vi "Stop Measurements.vi"(8 "error in (no error)":errorcluster, 11 "Pulse Controller in":refnum<class "Pulse Controller.lvclass">) -> (0 "error out":errorcluster, 3 "Pulse Controller out":refnum<class "Pulse Controller.lvclass">)   [LabVIEW 2016, in "Pulse Controller.lvclass"]
uses:
  Pulse Controller.lvclass
  C:/github/LabActor/Worker/Worker.lvclass
  C:/github/LabActor/Controllers/Process Controller/Process Controller.lvclass
  C:/github/LabActor/Template Module/Template Module.lvclass
  Worker/Worker.lvclass/Worker.ctl
  Process Controller/Process Controller.lvclass/Process Controller.ctl
  NHMFL_Core/Libraries/Instruments/Results/File Path Result/File Path Result.lvclass
  C:/github/NHMFL_Core/Libraries/Instruments/Results/Acquired Result/Acquired Result.lvclass
  Template Module/Template Module.lvclass/Template Module.ctl
  NHMFL_Core/Libraries/Instruments/Results/Acquired Result/Acquired Result.lvclass/Acquired Result.ctl
  Template Module/Read tdms stream.vi
  Template Module/Read Name.vi
  NHMFL_Core/Libraries/Instruments/Results/Acquired Result/Write Sender.vi
  Template Module/Read Reply to.vi
  Template Module/Read State.vi
  Process Controller/Read Awaiting Results.vi
  Read Pulse Controller Configuration.vi
  Template Module Messages/Result Reply Msg/Result Reply Msg.lvclass
  Process Controller/Process Controller.lvclass
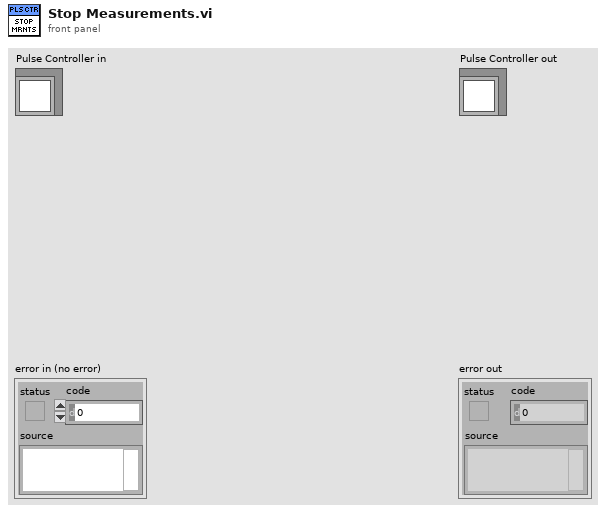
[diagram p1: front panel]
types:
  T1 = typedef "Worker State.ctl" = enum16{"Idle", "Starting", "Working", "Stopping"}
  T2 = typedef "Pulse Controller Configuration.ctl" = cluster{"Pre-trigger duration":dbl, "Post-trigger duration":dbl, "Open plot after pulse":bool}
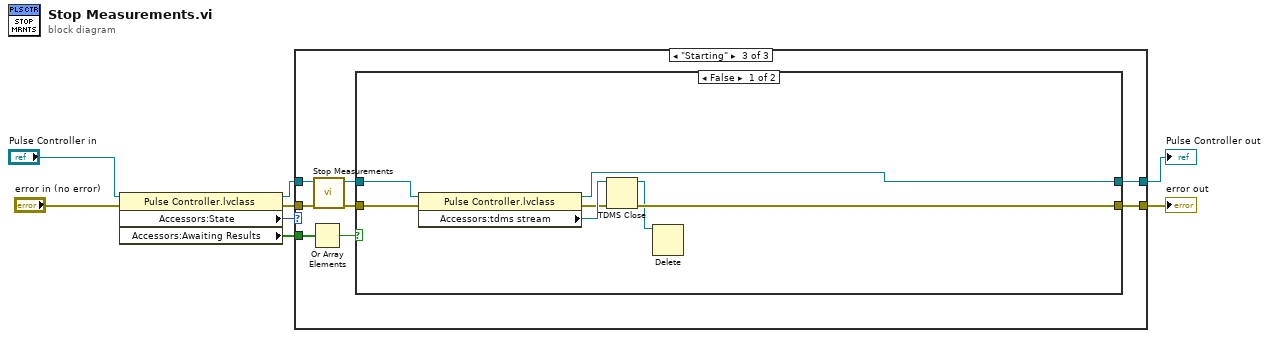
[diagram p0: block diagram]
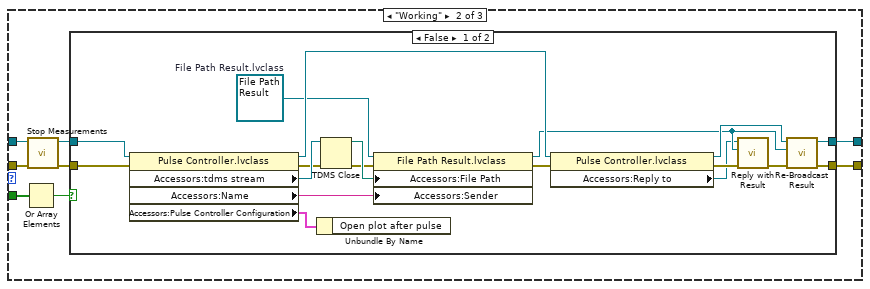
[diagram p3: hidden frame]
diagram:
  n1 = property class="Pulse Controller.lvclass"(reference="Pulse Controller in", error in="error in (no error)") -> (reference out=w3:refnum<class "Pulse Controller.lvclass">, error out=w5:errorcluster, "Accessors:State"=w2:T1, "Accessors:Awaiting Results"=w1:bool[])
  n2 = case shown="\"Starting\"" w2 {
    tunnel: w3 -> [w9 w18 w46]
    tunnel: w5 -> [w10 w14 w42]
    tunnel: [w9 w17 w45] -> w7
    tunnel: [w10 w16 w44] -> w6
    tunnel: w1 -> [_ w12 w40]
    frame "Idle", Default {
    }
    frame "Working" {
      n3 = Or Array Elements(Boolean array=w12) -> (logical OR=w11:bool)
      n4 = call-parent "Stop Measurements.vi"("error in (no error)"=w14, "Measure Controller in"=w18) -> ("error out"=w13:errorcluster, "Measure Controller out"=w15:refnum<class "Pulse Controller.lvclass">)  [unwired: 8 in]
      n5 = case shown="False" w11 {
        tunnel: [w34 w38] -> w17
        tunnel: [w23 w37] -> w16
        tunnel: w15 -> [w21 w38]
        tunnel: w13 -> [w20 w37]
        frame False {
          w31 = refnum<class "File Path Result.lvclass"> refnum  # File Path Result.lvclass
          n6 = property class="Pulse Controller.lvclass"(reference=w21, error in=w20) -> (reference out=w32:refnum<class "Pulse Controller.lvclass">, error out=w35:errorcluster, "Accessors:tdms stream"=w36:refnum<k34>, "Accessors:Name"=w26:string, "Accessors:Pulse Controller Configuration"=w33:T2)
          n7 = Unbundle By Name(w33) -> ()  [unwired: 1 out]
          n8 = TDMS Close(8:w35, 11:w36) -> (0:w29:errorcluster, 3:w30:path)
          n9 = property class="File Path Result.lvclass"(reference=w31, error in=w29, "Accessors:File Path"=w30, "Accessors:Sender"=w26) -> (reference out=w22:refnum<class "File Path Result.lvclass">, error out=w28:errorcluster)
          n10 = property class="Pulse Controller.lvclass"(reference=w32, error in=w28) -> (reference out=w25:refnum<class "Pulse Controller.lvclass">, error out=w27:errorcluster, "Accessors:Reply to"=w19:refnum<class "Result Reply Msg.lvclass">)
          n11 = call-dynamic "Reply with Result.vi"("error in (no error)"=w27, "Result"=w22, "Result Reply Msg in"=w19) -> ("error out"=w24:errorcluster)  [unwired: 7 in, 1 out]
          n12 = call-dynamic "Re-Broadcast Result.vi"("error in (no error)"=w24, "Acquired Result.lvclass"=w22, "Measure Object in"=w25) -> ("error out"=w23:errorcluster, "Measure Object out"=w34:refnum<class "Pulse Controller.lvclass">)  [unwired: 7 in]
        }
        frame True {
        }
      }
    }
    frame "Starting" {
      n13 = Or Array Elements(Boolean array=w40) -> (logical OR=w39:bool)
      n14 = call-parent "Stop Measurements.vi"("error in (no error)"=w42, "Measure Controller in"=w46) -> ("error out"=w41:errorcluster, "Measure Controller out"=w43:refnum<class "Pulse Controller.lvclass">)  [unwired: 8 in]
      n15 = case shown="False" w39 {
        tunnel: [w51 w55] -> w45
        tunnel: [w50 w54] -> w44
        tunnel: w43 -> [w49 w55]
        tunnel: w41 -> [w48 w54]
        frame False {
          n16 = property class="Pulse Controller.lvclass"(reference=w49, error in=w48) -> (reference out=w51:refnum<class "Pulse Controller.lvclass">, error out=w52:errorcluster, "Accessors:tdms stream"=w53:refnum<k34>)
          n17 = TDMS Close(8:w52, 11:w53) -> (0:w50:errorcluster, 3:w47:path)
          n18 = Delete(path (use dialog)=w47) -> ()  [unwired: 4 in, 3 out]
        }
        frame True {
        }
      }
    }
  }
  "error out" <- w6
  "Pulse Controller out" <- w7
